vi "Load New Bitfile.vi"(8 "error in (no error)":errorcluster, 10 "NewVal":path, 11 "Item Ref in":T1 format="%.0x") -> (0 "error out":errorcluster, 3 "Section Ref out":T1 format="%.0x")   [LabVIEW 2019, in "FPGA Addon System Explorer.lvlib"]
uses:
  FPGA Addon System Explorer.lvlib
  <vilib>/NI VeriStand/Custom Device Tools/Custom Device Utility Library/Custom Device Utility Library.lvlib
  Addon Shared/Constants.vi
  Addon Shared/FPGA Addon Shared.lvlib
  <vilib>/NI VeriStand/Custom Device Tools/Custom Device Utility Library/NI VeriStand - Search for Item by GUID.vi
  Addon Shared/FG Action.ctl
  <vilib>/NI VeriStand/Custom Device API/Custom Device API.lvlib
  <vilib>/NI VeriStand/Custom Device API/Custom Device Item Ref.ctl
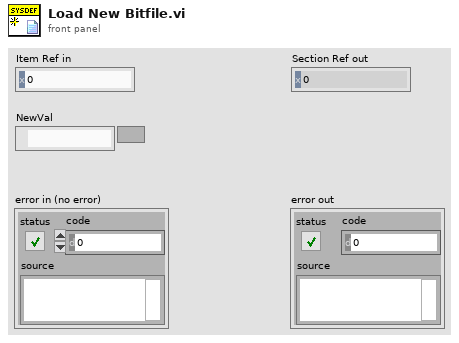
[diagram p1: front panel]
types:
  T1 = typedef "Custom Device API.lvlib/Custom Device Item Ref.ctl" = u64
  T2 = typedef "FPGA Addon Shared.lvlib/FG Action.ctl" = enum8{"GET", "SET"}
  T3 = typedef "Fifo_DMA_Config.ctl" = cluster{"Name":string, "Depth":u32, "Write? (Deprecated:Use Implementation)":bool, "Physical Channel":u32, "Base Address":u32, "Data Width":u32, "Data Type":T4, "FXP Properties":variant, "Write Window Address":u32, "Implementation":T5, "Control Set":u32}
  T4 = typedef "niFpgaDataTypeControl.ctl" = enum32{"Boolean", "I8", "I16", "I32", "I64", "U8", "U16", "U32", "U64", "FXP", "CustomControl", "SGL"}
  T5 = typedef "niFpgaDmaChannelImplementation.ctl" = enum16{"niFpgaTargetToHost", "niFpgaHostToTarget", "niFpgaPeerToPeerWriter", "niFpgaPeerToPeerReader", "niCoreTargetToHost", "niCoreHostToTarget"}
  T6 = typedef "niFpgaBitfileStructure_VI.ctl" = cluster{"Name":string, "RegisterMap":T7[], "Icon":T12}
  T7 = typedef "nirviControlStructure.ctl" = cluster{"Name":string, "Hidden":bool, "Indicator":bool, "Flattened Type":string, "Grouping":cluster{"Grouped":bool, "Member Names":string[], "Member IDs":u32[]}, "Address":u32, "Size":u32, "Class":u32, "Internal":bool, "Typedef":T8, "ID":u32, "Bidirectional":bool, "Synchronous":bool, "Mechanical Action":T9, "Sub Controls":T10[], "Access May Timeout":bool, "Register Node":bool}
  T8 = typedef "nirviTypdefDescription.ctl" = cluster{"Typedef":bool, "Path":path}
  T9 = typedef "nirviMechanicalAction.ctl" = enum8{"Switch When Pressed", "Switch When Released", "Switch Until Released", "Latch When Pressed", "Latch When Released", "Latch Until Released"}
  T10 = typedef "nirviSubControlStructure.ctl" = cluster{"Name":string, "flattened Type":string, "Cluster Information":T11, "Typedef":T8}
  T11 = typedef "nirviClusterElementControl.ctl" = cluster{"Name Hierarchy":string[], "Item Order":u32[]}
  T12 = typedef "imagedata.ctl" = cluster{"image type":i32, "image depth":i32, "image":u8[], "mask":u8[], "colors":u32[], "Rectangle":cluster{"left":i16, "top":i16, "right":i16, "bottom":i16}}
  T13 = typedef "FPGA Addon Shared.lvlib/Register Information.ctl" = cluster{"Name":string, "Data Type":T14, "Default Value":variant}
  T14 = typedef "FPGA Addon Shared.lvlib/Data Type.ctl" = enum8{"<Null>", "I8", "I16", "I32", "I64", "U8", "U16", "U32", "U64", "SGL", "Boolean", "Analog PWM In Settings", "Analog PWM In", "Digital PWM In Settings", "Digital PWM In", "Digital PWM Out", "Sine Out", "FXP+/-24.5", "FXP+/-16.5", "FXP+/-32.8", "FXP+/-64.32", "FXP+/-16.7", "FXP+/-20.5", "FXP+/-27.5", "FXP+/-32.16", "FXP +16.3", "FXP +18.3", "Digital Static In", "Digital Static Out", "Digital Static In Settings", "Digital WSS Out", "Quad Encoder Settings", "Quad Encoder In"}
  T15 = typedef "FPGA Addon Shared.lvlib/DMA Information.ctl" = cluster{"Name":string, "Data Type":T14}
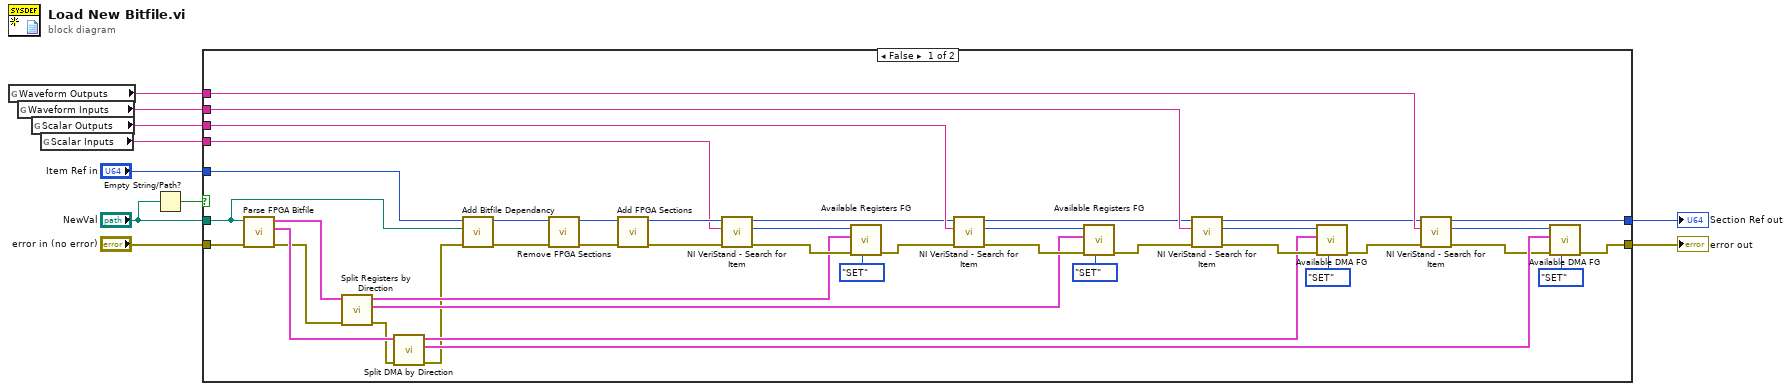
[diagram p0: block diagram]
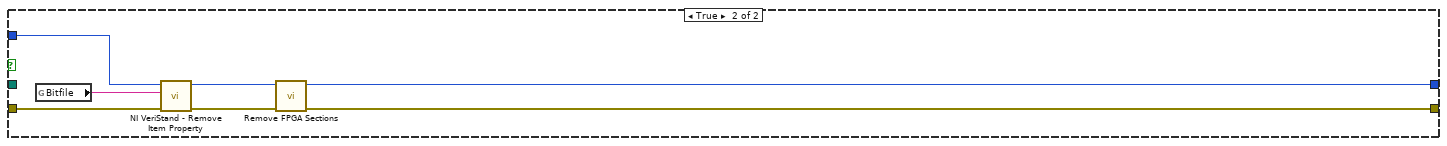
[diagram p2: hidden frame]
diagram:
  n1 = global read "Constants.vi" "Waveform Outputs"() -> (w7:string)
  n2 = global read "Constants.vi" "Waveform Inputs"() -> (w8:string)
  n3 = global read "Constants.vi" "Scalar Outputs"() -> (w9:string)
  n4 = global read "Constants.vi" "Scalar Inputs"() -> (w10:string)
  n5 = Empty String/Path?(string/path="NewVal") -> (empty?=w4:bool)
  n6 = case shown="False" w4 {
    tunnel: "NewVal" -> [w18 _]
    tunnel: "error in (no error)" -> [w52 w54]
    tunnel: w10 -> [w47 _]
    tunnel: w9 -> [w44 _]
    tunnel: w8 -> [w40 _]
    tunnel: w7 -> [w39 _]
    tunnel: [w24 w59] -> w6
    tunnel: [w22 w58] -> w5
    tunnel: "Item Ref in" -> [w17 w56]
    frame False {
      n7 = call "Parse FPGA Bitfile.vi"("error in (no error)"=w52, "Path"=w18) -> ("error out"=w13:errorcluster, "DMA configuration array"=w46:T3[], "vi info"=w45:T6)  [unwired: 7 in]
      n8 = call "Split Registers by Direction.vi"("error in"=w13, "vi info"=w45) -> ("error out"=w12:errorcluster, "Controls"=w14:T13[], "Indicator"=w15:T13[])  [unwired: 7 in]
      n9 = call "Split DMA by Direction.vi"("error in"=w12, "DMA configuration array"=w46) -> ("error out"=w11:errorcluster, "HostToTarget"=w26:T15[], "TargetToHost"=w31:T15[])  [unwired: 7 in]
      n10 = call "Add Bitfile Dependancy.vi"("error in (no error)"=w11, "Path"=w18, "Item Ref in"=w17) -> ("error out"=w19:errorcluster, "Item Ref out"=w16:T1)  [unwired: 7 in]
      n11 = call "Remove FPGA Sections.vi"("error in (no error)"=w19, "Item Ref in"=w16) -> ("error out"=w20:errorcluster, "Item Ref out"=w21:T1)  [unwired: 8 in]
      n12 = call "Add FPGA Sections.vi"("error in (no error)"=w20, "Node Ptr"=w21) -> ("error out"=w50:errorcluster, "Parent Ref out"=w51:T1)  [unwired: 8 in]
      n13 = call-poly <vilib>:"NI VeriStand - Search for Item.vi"("error in"=w50, "Item GUID"=w47, "Section Ref in"=w51) -> ("error out"=w49:errorcluster, "Item Ref"=w48:T1, "Section Ref out"=w42:T1)  [unwired: 5 in, 1 out]
      n14 = call "Available Registers FG.vi"("Action"=FG_Action."SET", "error in (no error)"=w49, "Available Registers"=w15, "Item Ref"=w48) -> ("error out"=w43:errorcluster)  [unwired: 5 in, 2 out]
      n15 = call-poly <vilib>:"NI VeriStand - Search for Item.vi"("error in"=w43, "Item GUID"=w44, "Section Ref in"=w42) -> ("error out"=w35:errorcluster, "Item Ref"=w34:T1, "Section Ref out"=w38:T1)  [unwired: 5 in, 1 out]
      n16 = call "Available Registers FG.vi"("Action"=FG_Action."SET", "error in (no error)"=w35, "Available Registers"=w14, "Item Ref"=w34) -> ("error out"=w33:errorcluster)  [unwired: 5 in, 2 out]
      n17 = call-poly <vilib>:"NI VeriStand - Search for Item.vi"("error in"=w33, "Item GUID"=w40, "Section Ref in"=w38) -> ("error out"=w32:errorcluster, "Item Ref"=w41:T1, "Section Ref out"=w28:T1)  [unwired: 5 in, 1 out]
      n18 = call "Available DMA FG.vi"("Action"=FG_Action."SET", "error in (no error)"=w32, "Available DMA"=w31, "Item Ref"=w41) -> ("error out"=w29:errorcluster)  [unwired: 5 in, 2 out]
      n19 = call-poly <vilib>:"NI VeriStand - Search for Item.vi"("error in"=w29, "Item GUID"=w39, "Section Ref in"=w28) -> ("error out"=w25:errorcluster, "Item Ref"=w27:T1, "Section Ref out"=w22:T1)  [unwired: 5 in, 1 out]
      n20 = call "Available DMA FG.vi"("Action"=FG_Action."SET", "error in (no error)"=w25, "Available DMA"=w26, "Item Ref"=w27) -> ("error out"=w24:errorcluster)  [unwired: 5 in, 2 out]
    }
    frame True {
      n21 = global read "Constants.vi" "Bitfile"() -> (w57:string)
      n22 = call <vilib>:"NI VeriStand - Remove Item Property.vi"("error in (no error)"=w54, "Property Name"=w57, "Item Ref in"=w56) -> ("error out"=w53:errorcluster, "Item Ref out"=w55:T1)  [unwired: 6 in, 1 out]
      n23 = call "Remove FPGA Sections.vi"("error in (no error)"=w53, "Item Ref in"=w55) -> ("error out"=w59:errorcluster, "Item Ref out"=w58:T1)  [unwired: 8 in]
    }
  }
  "error out" <- w6
  "Section Ref out" <- w5
